vi "execute.vi"(10 "task token":refnum<class "null task token.lvclass">, 11 "call by reference action in":refnum<class "call by reference action.lvclass">) -> (3 "result":refnum<class "result.lvclass">)   [LabVIEW 2013, in "call by reference action.lvclass"]
uses:
  call by reference action.lvclass
  result/result.lvclass
  task token/null task token.lvclass
  call by reference action.lvclass/call by reference action.ctl
  action/action.lvclass/action.ctl
  action/action.lvclass
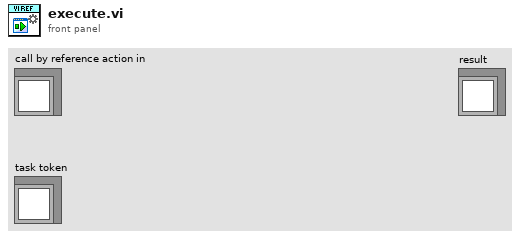
[diagram p1: front panel]
types:
  T1 = typedef "call by reference action.lvclass/function definition.ctl" = refnum<vi>
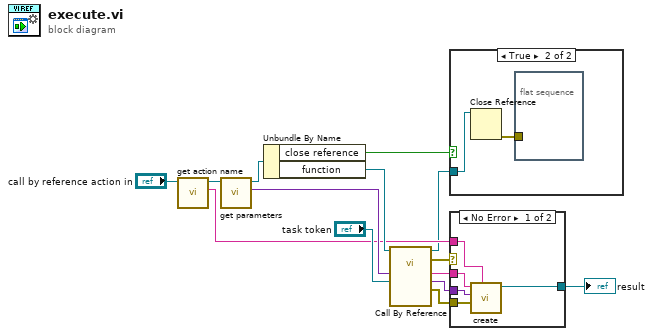
[diagram p0: block diagram]
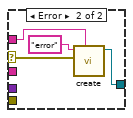
[diagram p3: hidden frame]
diagram:
  n1 = call "get action name.vi"("action in"="call by reference action in") -> ("action name"=w7:string, "action out"=w8:refnum<class "call by reference action.lvclass">)  [unwired: 9 in]
  n2 = call "get parameters.vi"("action in"=w8) -> ("parameters"=w10:variant, "action out"=w11:refnum<class "call by reference action.lvclass">)  [unwired: 9 in]
  n3 = Unbundle By Name(w11) -> ("close reference"=w2:bool, "function"=w13:T1)
  n4 = call-by-ref "?"(reference=w13, "task token"="task token", "parameters"=w10) -> (reference out=w1:T1, error out=w6:errorcluster, "error"=w3:errorcluster, "data"=w4:variant, "data ID"=w5:string)  [unwired: 8 in]
  n5 = case shown="True" w2 {
    tunnel: w1 -> [_ w16]
    frame False {
    }
    frame True {
      n6 = Close Reference(reference=w16) -> (error out=w15:errorcluster)  [unwired: 1 in]
      n7 = flat-sequence {
        tunnel: w15 -> [_]
        frame #0 {
        }
      }
    }
  }
  n8 = case shown="No Error" w6 {
    selector: w6 -> [_ w23]
    tunnel: [w21 w22] -> w9
    tunnel: w7 -> [w20 w24]
    tunnel: w5 -> [w19 _]
    tunnel: w4 -> [w18 _]
    tunnel: w3 -> [w17 _]
    frame No Error {
      n9 = call "create.vi"("generating action"=w20, "error"=w17, "data"=w18, "data ID"=w19) -> ("result out"=w21:refnum<class "result.lvclass">)  [unwired: 7 in]
    }
    frame Error {
      n10 = call "create.vi"("generating action"=w24, "data"=w23, "data ID"="error") -> ("result out"=w22:refnum<class "result.lvclass">)  [unwired: 8 in]
    }
  }
  "result" <- w9
